vi "Examples FitImageToContainer.vi"() -> ()   [LabVIEW 2020, in "LcPictureBox.lvclass"]
uses:
  LcPictureBox.lvclass
  System.Windows.Forms
  <extravilib>/ChannelInstances/Event Messenger-c(bool,i32,str)/Instantiate.vi
  <extravilib>/ChannelInstances/Event Messenger-c(bool,i32,str)/))Channel.vi
  <extravilib>/ChannelInstances/Event Messenger-c(bool,i32,str).lvlib
  <vilib>/picture/picture.llb/imagedata.ctl
panel:
  in  "LeftPictureBox":refnum<k24>(container)
  in  "RightPictureBox":refnum<k24>(container)
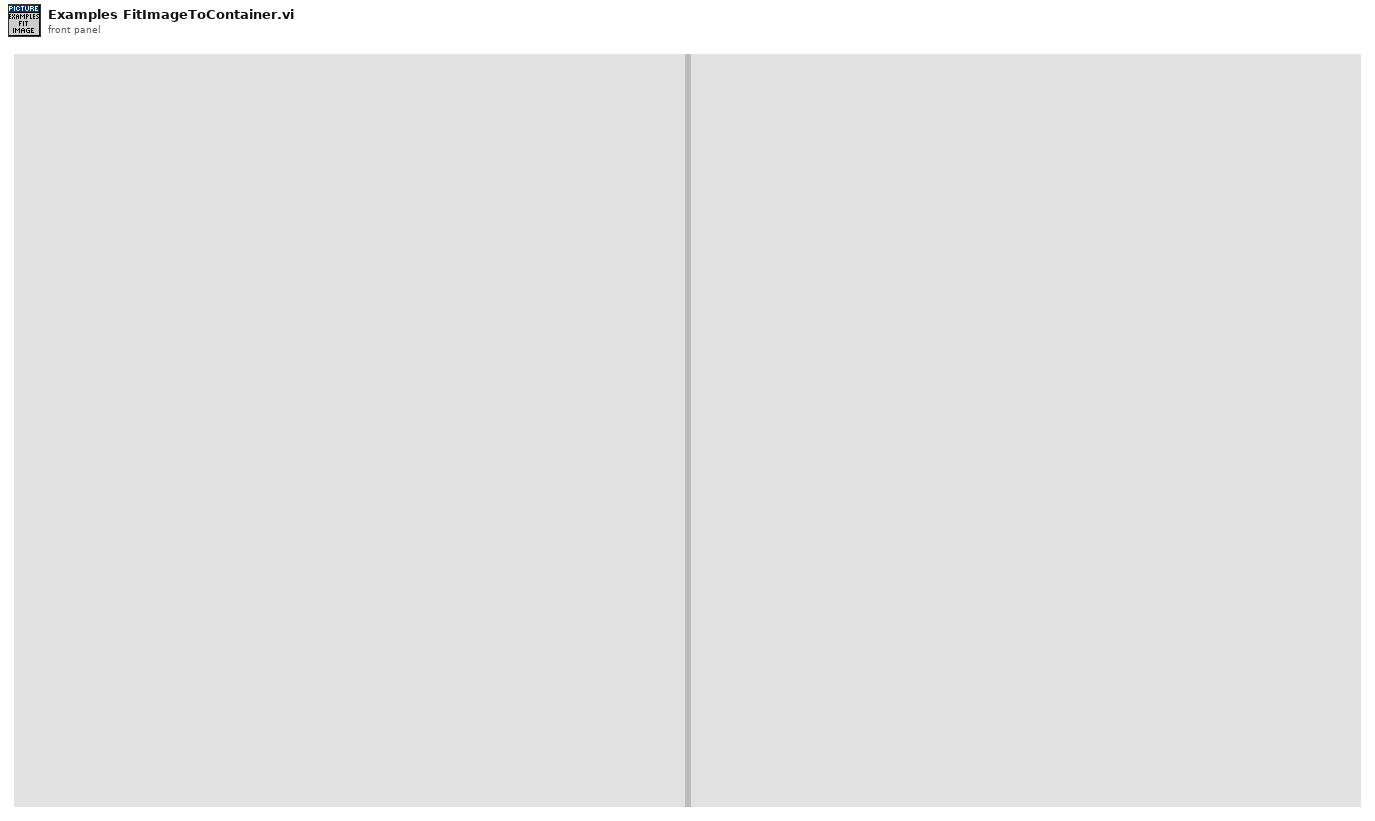
[diagram p1: front panel]
types:
  T1 = typedef "imagedata.ctl" = cluster{"image type":i32, "image depth":i32, "image":u8[], "mask":u8[], "colors":u32[], "Rectangle":cluster{"left":i16, "top":i16, "right":i16, "bottom":i16}}
  T2 = typedef "Event Messenger-c(bool,i32,str).lvlib/))Channel.ctl" = refnum<queue>
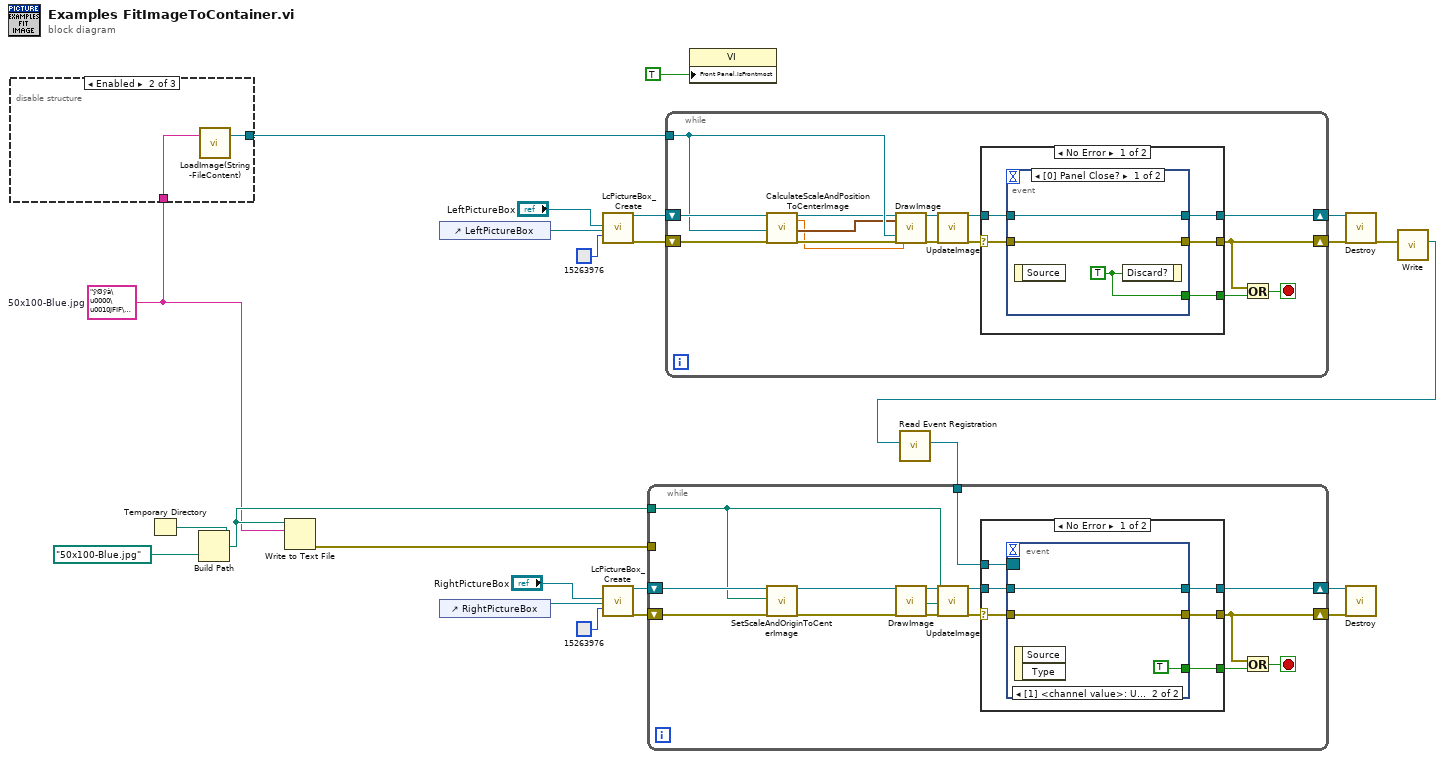
[diagram p0: block diagram]
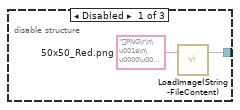
[diagram p2: hidden frame]
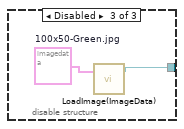
[diagram p3: hidden frame]
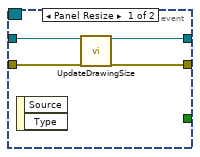
[diagram p4: hidden frame]
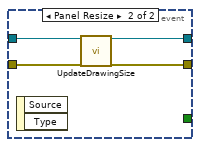
[diagram p6: hidden frame]
diagram:
  w1 = "ÿØÿà\u0000\u0010JFIF\u0000\u0001\u0001\u0001\u0000`\u0000`\u0000\u0000ÿá\u0000fExif\u0000\u0000MM\u0000*\u0000\u0000\u0000\b\u0000\u0006\u0001\u0012\u0000\u0003\u0000\u0000\u0000\u0001\u0000\u0001\u0000\u0000\u0003\u0001\u0000\u0005\u0000\u0000\u0000\u0001\u0000\u0000\u0000V\u0003\u0003\u0000\u0001\u0000\u0000\u0000\u0001\u0000\u0000\u0000\u0000Q\u0010\u0000\u0001\u0000\u0000\u0000\u0001\u0001\u0000\u0000\u0000Q\u0011\u0000\u0004\u0000\u0000\u0000\u0001\u0000\u0000\u000eÃQ\u0012\u0000\u0004\u0000\u0000\u0000\u0001\u0000\u0000\u000eÃ\u0000\u0000\u0000\u0000\u0000\u0001 \u0000\u0000±ÿÛ\u0000C\u0000\u0002\u0001\u0001\u0002\u0001\u0001\u0002\u0002\u0002\u0002\u0002\u0002\u0002\u0002\u0003\u0005\u0003\u0003\u0003\u0003\u0003\u0006\u0004\u0004\u0003\u0005\u0007\u0006\u0007\u0007\u0007\u0006\u0007\u0007\b\t\u000b\t\b\b\n\b\u0007\u0007\n\r\n\n\u000b\f\f\f\f\u0007\t\u000e\u000f\r\f\u000e\u000b\f\f\fÿÛ\u0000C\u0001\u0002\u0002\u0002\u0003\u0003\u0003\u0006\u0003\u0003\u0006\f\b\u0007\b\f\f\f\f\f\f\f\f\f\f\f\f\f\f\f\f\f\f\f\f\f\f\f\f\f\f\f\f\f\f\f\f\f\f\f\f\f\f\f\f\f\f\f\f\f\f\f\f\f\fÿÀ\u0000\u0011\b\u0000d\u00002\u0003\u0001\"\u0000\u0002\u0011\u0001\u0003\u0011\u0001ÿÄ\u0000\u001f\u0000\u0000\u0001\u0005\u0001\u0001\u0001\u0001\u0001\u0001\u0000\u0000\u0000\u0000\u0000\u0000\u0000\u0000\u0001\u0002\u0003\u0004\u0005\u0006\u0007\b\t\n\u000bÿÄ\u0000µ\u0010\u0000\u0002\u0001\u0003\u0003\u0002\u0004\u0003\u0005\u0005\u0004\u0004\u0000\u0000\u0001}\u0001\u0002\u0003\u0000\u0004\u0011\u0005\u0012!1A\u0006\u0013Qa\u0007\"q\u00142¡\b#B±Á\u0015RÑð$3br\t\n\u0016\u0017\u0018\u0019\u001a%&'()*456789:CDEFGHIJSTUVWXYZcdefghijstuvwxyz¢£¤¥¦§¨©ª²³´µ¶·¸¹ºÂÃÄÅÆÇÈÉÊÒÓÔÕÖ×ØÙÚáâãäåæçèéêñòóôõö÷øùúÿÄ\u0000\u001f\u0001\u0000\u0003\u0001\u0001\u0001\u0001\u0001\u0001\u0001\u0001\u0001\u0000\u0000\u0000\u0000\u0000\u0000\u0001\u0002\u0003\u0004\u0005\u0006\u0007\b\t\n\u000bÿÄ\u0000µ\u0011\u0000\u0002\u0001\u0002\u0004\u0004\u0003\u0004\u0007\u0005\u0004\u0004\u0000\u0001\u0002w\u0000\u0001\u0002\u0003\u0011\u0004\u0005!1\u0006\u0012AQ\u0007aq\u0013\"2\b\u0014B¡±Á\t#3Rð\u0015brÑ\n\u0016$4á%ñ\u0017\u0018\u0019\u001a&'..."  # 50x100-Blue.jpg
  n1 = disable-structure shown="Enabled" {
    disable-tunnel: [w25 w28 w29] -> w2
    disable-tunnel: w1 -> [_ w27 _]
    frame Disabled {
      w26 = "PNG\r\n\u001a\n\u0000\u0000\u0000\rIHDR\u0000\u0000\u00002\u0000\u0000\u00002\b\u0006\u0000\u0000\u0000\u001e?±\u0000\u0000\u0000\u0001sRGB\u0000®Î\u001cé\u0000\u0000\u0000\u0004gAMA\u0000\u0000±\u000büa\u0005\u0000\u0000\u0000\tpHYs\u0000\u0000\u000eÄ\u0000\u0000\u000eÄ\u0001+\u000e\u001b\u0000\u0000\u0002IDAThCí1kÛ@\u0018ß\u0016I\bä\u0018Å\u0016M\u0003b\u001a:tþA¡¦ £Wgèbºeö¥C¼zÌÖ©dÈ?ÈÞ¡¤ ­p\"ú°\u0005íw§S­Z\u0004Û­k¸\u0007ÌY§;½zï¾ï;\u001fÝ´ö~â\u0001ðX¶ÿ=Újh#ª¡¨6¢\u001aÚjh#ª¡¨6¢\u001aÚj³§1:_'¸9]o\u000fÇ¶¼ ÆIÃÉ\u001cg£ëîà¸f«µ¨Xçþ\u001d±êè:Ï\u000bCösèáûüá4fàyèZ\tFñ\u0015:Ó¹\u001c°\u0001\u0015éw&7iòòÊ,c\u0018^áhVÇië\t^>~p\u0011}+¨Xgó\u001cI\u0019>Ì¨uÂ\u001c¼qx;ÃeJá0\rÐ\f.Ñ¸ËÉûÖÞµ5tS>\u001b\u0018MèEøË\u0004\u0001úIAîóxõM+»<7ù²&øL\u0002íÚ\u000e\u0006ü60\u0014\fïãÂÈÃï*twÄ¨QBíâbràØðiÒh²iüè5<1÷è;Ãù4¢p°1h¸hË\u0011Õè,(\u0019iÛ.U\u0005ÚNj{Û-=å/\u0004\\ü`\u0018gCÖÃpqâÒê±k\u001cÐnøTmzD®LG²:G\f\u0013/åWaeó,4r¾Ì)thÕÿ¨:ð:«¤s|â­ifa\u000b2\n\u0019Þ\n\u0018>ò¼¶jx\u000bÐ9qÈóÂÙ¥Ð¡\u0017¿É|¹¿ÕG\u0001:QaB\u001f..."  # 50x50_Red.png
      n2 = call "LoadImage(String-FileContent).vi"("ImageFileContent"=w26) -> ("ImageOut"=w25:refnum<k24>)  [unwired: 16 in, 2 out]
    }
    frame Enabled {
      n3 = call "LoadImage(String-FileContent).vi"("ImageFileContent"=w27) -> ("ImageOut"=w28:refnum<k24>)  [unwired: 16 in, 2 out]
    }
    frame Disabled {
      w30 = T1 {"image type"=0, "image depth"=24, "image"=array[15000 elements], "mask"=[], "colors"=[], "Rectangle"={"left"=0, "top"=0, "right"=100, "bottom"=50}}  # 100x50-Green.jpg
      n4 = call "LoadImage(ImageData).vi"("image data"=w30) -> ("ImageOut"=w29:refnum<k24>)  [unwired: 16 in, 2 out]
    }
  }
  n5 = Temporary Directory() -> (w16:path)
  n6 = Build Path(base path=w16, name or relative path=path "50x100-Blue.jpg" ("Filename")) -> (appended path=w7:path)
  n7 = Write to Text File(file (use dialog)=w7, text=w1) -> (error out=w6:errorcluster)  [unwired: 2 in, 2 out]
  n8 = control-ref of="LeftPictureBox"() -> (w23:refnum<vi>)
  n9 = control-ref of="RightPictureBox"() -> (w9:refnum<vi>)
  n10 = call "LcPictureBox_Create.vi"("PictureBox"="LeftPictureBox", "PictureBoxActiveXReference"=w23, "BgColor(None)"=u32 15263976) -> ("reference out"=w18:refnum<class "LcPictureBox.lvclass">, "Error Out"=w17:errorcluster)  [unwired: 14 in, 1 out]
  n11 = call "LcPictureBox_Create.vi"("PictureBox"="RightPictureBox", "PictureBoxActiveXReference"=w9, "BgColor(None)"=u32 15263976) -> ("reference out"=w13:refnum<class "LcPictureBox.lvclass">, "Error Out"=w14:errorcluster)  [unwired: 14 in, 1 out]
  n12 = while {
    tunnel: w2 -> [w35]
    shift-right: [w45] -> w21
    shift-left: w18 -> [w37]
    shift-right: [w42] -> w19
    shift-left: w17 -> [w36]
    stop <- w40 stop-if-true
    n13 = call-dynamic "CalculateScaleAndPositionToCenterImage.vi"("reference in"=w37, "Image"=w35, "Error In"=w36) -> ("reference out"=w34:refnum<class "LcPictureBox.lvclass">, "ScaleFactor"=w31:sgl, "ImagePosition"=w32:cluster{"x":sgl, "y":sgl}, "Error Out"=w33:errorcluster)  [unwired: 13 in]
    n14 = call-dynamic "DrawImage.vi"("reference in"=w34, "UpperLeftCorner(0,0)"=w32, "Image"=w35, "Error In"=w33, "ScaleFactor(1)"=w31) -> ("reference out"=w39:refnum<class "LcPictureBox.lvclass">, "Error Out"=w38:errorcluster)  [unwired: 13 in]
    n15 = call-dynamic "UpdateImage.vi"("reference in"=w39, "Error In"=w38) -> ("reference out"=w43:refnum<class "LcPictureBox.lvclass">, "Error Out"=w44:errorcluster)  [unwired: 14 in, 2 out]
    n16 = case shown="No Error" w44 {
      selector: w44 -> [w50 w59]
      tunnel: w43 -> [w49 w58]
      tunnel: [w48 w59] -> w42
      tunnel: [w47 w58] -> w45
      tunnel: [w46 _] -> w41
      frame No Error {
        n17 = event shown="[0] Panel Close?" {
          selector: _ -> [_ _]
          dyn-events: _ -> [_ _]
          timeout: _ -> [_ _]
          tunnel: w50 -> [w53 w56]
          tunnel: [w53 w54] -> w48
          tunnel: w49 -> [w52 w57]
          tunnel: [w52 w55] -> w47
          tunnel: [w51 _] -> w46
          event Panel Close? {
            w51 = TRUE ("Discard?")
            n18 = event-data() -> ()  [unwired: 1 in, 1 out]
            n19 = event-data("Discard?"=w51) -> ()  [unwired: 1 in, 1 out]
          }
          event Panel Resize {
            n20 = event-data() -> ()  [unwired: 1 in, 2 out]
            n21 = call-dynamic "UpdateDrawingSize.vi"("reference in"=w57, "Error In"=w56) -> ("reference out"=w55:refnum<class "LcPictureBox.lvclass">, "Error Out"=w54:errorcluster)  [unwired: 16 in]
          }
        }
      }
      frame Error {
      }
    }
    n22 = Or(x=w42, y=w41) -> (x .or. y?=w40:bool)
  }
  n23 = property class="VI"("Front Panel.IsFrontmost"=TRUE ("Front Panel Window:Is Frontmost")) -> ()  [unwired: 2 in, 2 out]
  n24 = call-dynamic "Destroy.vi"("reference in"=w21, "Error In"=w19) -> ("Error Out"=w5:errorcluster)  [unwired: 16 in, 1 out]
  n25 = call <extravilib>:"Write.vi"("element"=w5) -> ("channel"=w3:T2)  [unwired: 9 in, 1 out]
  n26 = call <extravilib>:"Read Event Registration.vi"("channel"=w3) -> ("event registration refnum"=w4:refnum<event-registration>)  [unwired: 10 in]
  n27 = while {
    tunnel: w7 -> [w63]
    shift-right: [w73] -> w11
    shift-left: w13 -> [w65]
    shift-right: [w70] -> w12
    shift-left: w14 -> [w64]
    tunnel: w6 -> [_]
    tunnel: w4 -> [w62]
    stop <- w68 stop-if-true
    n28 = call-dynamic "SetScaleAndOriginToCenterImage.vi"("reference in"=w65, "ImageFile"=w63, "Error In"=w64) -> ("reference out"=w60:refnum<class "LcPictureBox.lvclass">, "Error Out"=w61:errorcluster)  [unwired: 13 in, 2 out]
    n29 = call-dynamic "DrawImage.vi"("reference in"=w60, "Filename"=w63, "Error In"=w61) -> ("reference out"=w67:refnum<class "LcPictureBox.lvclass">, "Error Out"=w66:errorcluster)  [unwired: 15 in]
    n30 = call-dynamic "UpdateImage.vi"("reference in"=w67, "Error In"=w66) -> ("reference out"=w71:refnum<class "LcPictureBox.lvclass">, "Error Out"=w72:errorcluster)  [unwired: 14 in, 2 out]
    n31 = case shown="No Error" w72 {
      selector: w72 -> [w79 w88]
      tunnel: w71 -> [w78 w87]
      tunnel: [w77 w88] -> w70
      tunnel: [w76 w87] -> w73
      tunnel: [w74 _] -> w69
      tunnel: w62 -> [w75 _]
      frame No Error {
        n32 = event shown="[1] <channel value>: User Event" {
          selector: w75 -> [_ _]
          dyn-events: _ -> [_ _]
          timeout: _ -> [_ _]
          tunnel: w79 -> [w82 w86]
          tunnel: [w80 w86] -> w77
          tunnel: w78 -> [w83 w85]
          tunnel: [w81 w85] -> w76
          tunnel: [_ TRUE] -> w74
          event Panel Resize {
            n33 = event-data() -> ()  [unwired: 1 in, 2 out]
            n34 = call-dynamic "UpdateDrawingSize.vi"("reference in"=w83, "Error In"=w82) -> ("reference out"=w81:refnum<class "LcPictureBox.lvclass">, "Error Out"=w80:errorcluster)  [unwired: 16 in]
          }
          event User Event {
            n35 = event-data() -> ()  [unwired: 1 in, 2 out]
          }
        }
      }
      frame Error {
      }
    }
    n36 = Or(x=w70, y=w69) -> (x .or. y?=w68:bool)
  }
  n37 = call-dynamic "Destroy.vi"("reference in"=w11, "Error In"=w12) -> ()  [unwired: 16 in, 2 out]
